vi "Stop.vi"(8 "error in (no error)":errorcluster, 11 "TimeStamper in":refnum<class "TimeStamper.lvclass">) -> (0 "error out":errorcluster, 3 "TimeStamper out":refnum<class "TimeStamper.lvclass">)   [LabVIEW 2010, in "TimeStamper.lvclass"]
uses:
  TimeStamper.lvclass
  TimeStamper.lvclass/TimeStamper.ctl
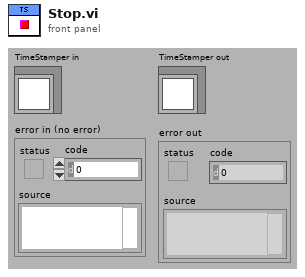
[diagram p1: front panel]
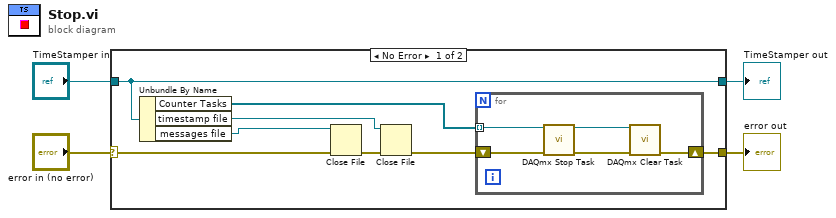
[diagram p0: block diagram]
diagram:
  n1 = case shown="No Error" "error in (no error)" {
    selector: "error in (no error)" -> [w6 w19]
    tunnel: [w11 w19] -> w1
    tunnel: [w10 w18] -> w2
    tunnel: "TimeStamper in" -> [w10 w18]
    frame No Error {
      n2 = Unbundle By Name(w10) -> ("Counter Tasks"=w12:refnum<k21>[], "timestamp file"=w9:refnum<file>, "messages file"=w8:refnum<file>)
      n3 = Close File(refnum=w8, error in=w6) -> (error out=w7:errorcluster)  [unwired: 1 out]
      n4 = Close File(refnum=w9, error in=w7) -> (error out=w5:errorcluster)  [unwired: 1 out]
      n5 = for {
        tunnel: w12 -> [w17] mode=indexing
        shift-right: [w13] -> w11
        shift-left: w5 -> [w14]
        n6 = call <vilib>:"DAQmx Stop Task.vi"("task/channels in"=w17, "error in"=w14) -> ("task out"=w16:refnum<k21>, "error out"=w15:errorcluster)  [unwired: 12 in]
        n7 = call <vilib>:"DAQmx Clear Task.vi"("task in"=w16, "error in"=w15) -> ("error out"=w13:errorcluster)  [unwired: 13 in]
      }
    }
    frame Error {
    }
  }
  "error out" <- w1
  "TimeStamper out" <- w2
